vi "Skew_Image3.vi"(4 "[IN] Skewed Image":T1, 5 "[IN] Share Angle":u16 max=89 step=1, 6 "[IN] Calculation mode":enum16{"Single core", "2x cores", "4x cores"}(ring), 7 "error IN":errorcluster, 8 "[IN] Y = Array rows":i32, 9 "[IN] X = Array cols":i32, 10 "[IN] Source Image U16":u16[][](array[numeric])) -> (0 "error OUT":errorcluster, 3 "[OUT] Skewed Image":T1)   [LabVIEW 2020]
uses:
  <vilib>/vision/Image Controls.llb/IMAQ Image.ctl
  <vilib>/vision/NI_Vision_Development_Module.lvlib
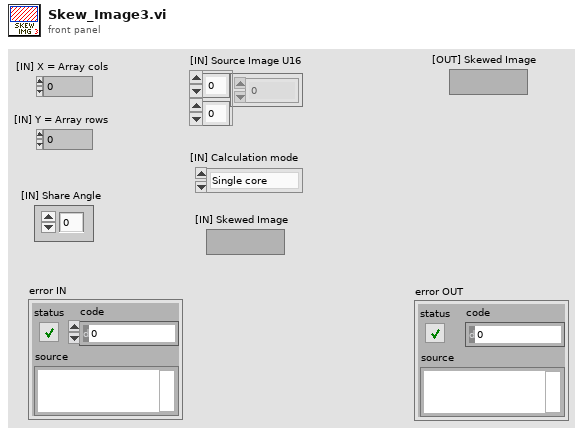
[diagram p1: front panel]
types:
  T1 = typedef "IMAQ Image.ctl" = refnum<image>
  T2 = typedef "Image Type" = u32
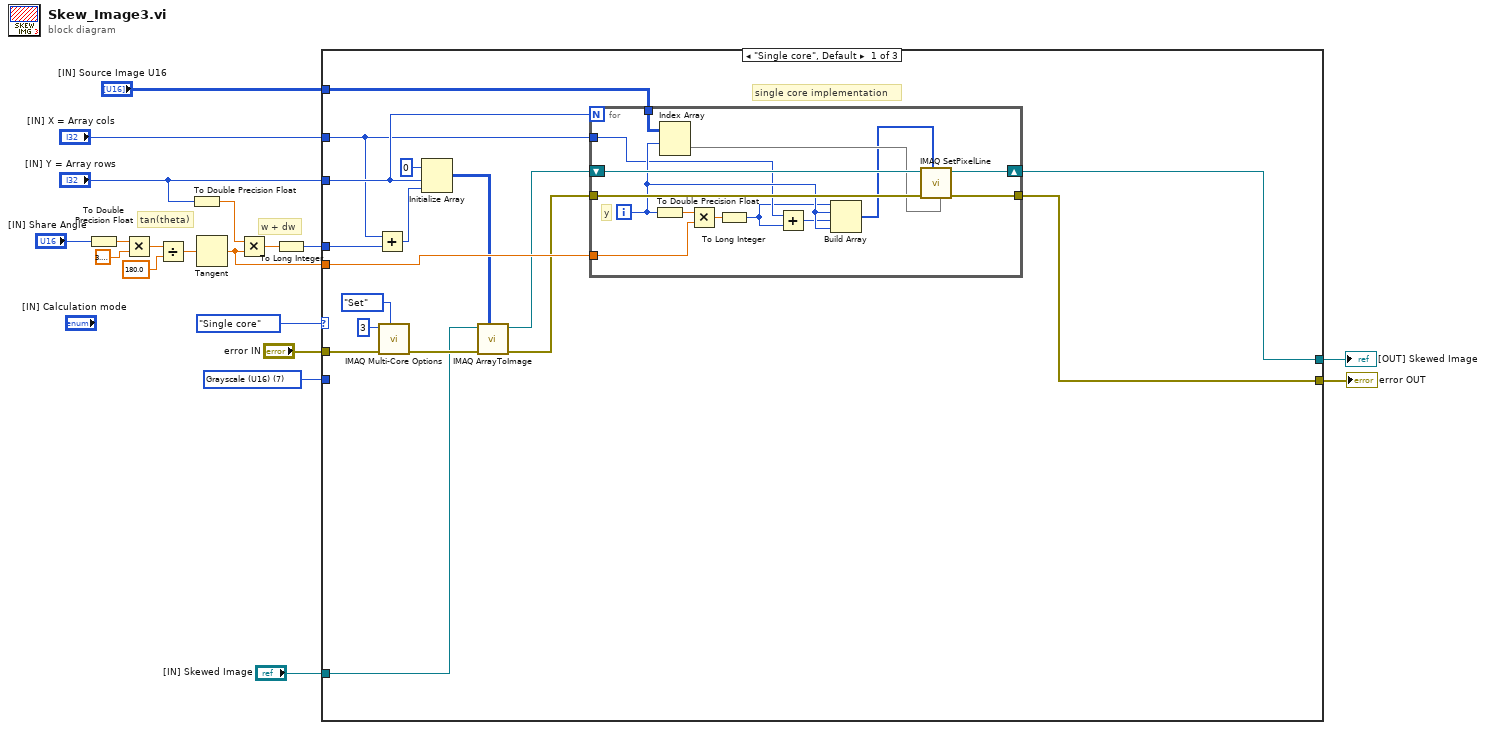
[diagram p0: block diagram]
diagram:
  w4 = T2 7 items=["Grayscale (U8)", "Grayscale (I16)", "Grayscale (SGL)", "Complex (CSG)", "RGB (U32)", "HSL (U32)", "RGB (U64)", "Grayscale (U16)"] ("Image Type")
  # "w + dw"
  # "tan(theta)"
  n1 = To Double Precision Float(number="[IN] Share Angle") -> (double precision float=w19:dbl)
  n2 = Multiply(x=w19, y=3.141592653589793) -> (x*y=w18:dbl)
  n3 = Divide(x=w18, y=180.0) -> (x/y=w16:dbl)
  n4 = To Double Precision Float(number="[IN] Y = Array rows") -> (double precision float=w10:dbl)
  n5 = Tangent(1:w16) -> (0:w14:dbl)
  n6 = Multiply(x=w10, y=w14) -> (x*y=w13:dbl)
  n7 = To Long Integer(number=w13) -> (32bit integer=w15:i32)
  n8 = case shown="\"Single core\", Default" enum16{"Single core", "2x cores", "4x cores"}."Single core" ("[IN] Calculation mode") {
    tunnel: w15 -> [w29 _ _]
    tunnel: w14 -> [w28 _ _]
    tunnel: "[IN] Source Image U16" -> [w31 _ _]
    tunnel: "[IN] X = Array cols" -> [w20 _ _]
    tunnel: "[IN] Y = Array rows" -> [w30 _ _]
    tunnel: "error IN" -> [w34 w51 w53]
    tunnel: [w21 w51 w53] -> w5
    tunnel: w4 -> [_ _ _]
    tunnel: [w22 w52 w54] -> w3
    tunnel: "[IN] Skewed Image" -> [w25 w52 w54]
    frame "Single core", Default {
      # "single core implementation"
      n9 = Add(x=w20, y=w29) -> (x+y=w32:i32)
      n10 = call "IMAQ Multi-Core Options"("Get/Set Number of Cores (Get)"=enum32{"Get", "Set", "Set Max Available"}."Set", "error in (no error)"=w34, "Specified Number of Cores"=u32 3) -> ("error out"=w27:errorcluster)  [unwired: 7 in, 1 out]
      n11 = Initialize Array(u16 0, w30, w32) -> (w26:u16[][])
      n12 = call "IMAQ ArrayToImage"("Image Pixels (U16)"=w26, "error in (no error)"=w27, "Image"=w25) -> ("error out"=w23:errorcluster, "Image Out"=w24:T1)  [unwired: 7 in]
      n13 = for {
        N: w30 -> [_]
        shift-right: [w44] -> w22
        shift-left: w24 -> [w46]
        tunnel: w31 -> [w50]
        tunnel: w28 -> [w48]
        tunnel: w20 -> [w38]
        tunnel: w23 -> [w45]
        tunnel: [w43] -> w21
        i -> [w40]
        # "y"
        n14 = To Double Precision Float(number=w40) -> (double precision float=w49:dbl)
        n15 = Index Array(array=w50, index (row)=w40) -> (element=w42:u16[])  [unwired: 1 in]
        n16 = Multiply(x=w49, y=w48) -> (x*y=w47:dbl)
        n17 = To Long Integer(number=w47) -> (32bit integer=w37:i32)
        n18 = Add(x=w38, y=w37) -> (x+y=w39:i32)
        n19 = Build Array(w37, w40, w39, w40) -> (w41:i32[])
        n20 = call "IMAQ SetPixelLine"("Pixels Line (U16)"=w42, "Line Coordinates"=w41, "error in (no error)"=w45, "Image"=w46) -> ("error out"=w43:errorcluster, "Image Out"=w44:T1)  [unwired: 6 in]
      }
    }
    frame "2x cores" {
    }
    frame "4x cores" {
    }
  }
  "error OUT" <- w5
  "[OUT] Skewed Image" <- w3
